vi "Read Value.vi"(8 "error in (no error)":errorcluster, 11 "sfixed32 in":refnum<class "sfixed32.lvclass">) -> (0 "error out":errorcluster, 2 "Value":i32, 3 "sfixed32 out":refnum<class "sfixed32.lvclass">)   [LabVIEW 2020, in "Protobuf RAW.lvlib" / "sfixed32.lvclass"]
uses:
  sfixed32.lvclass
  sfixed32.lvclass/sfixed32.ctl
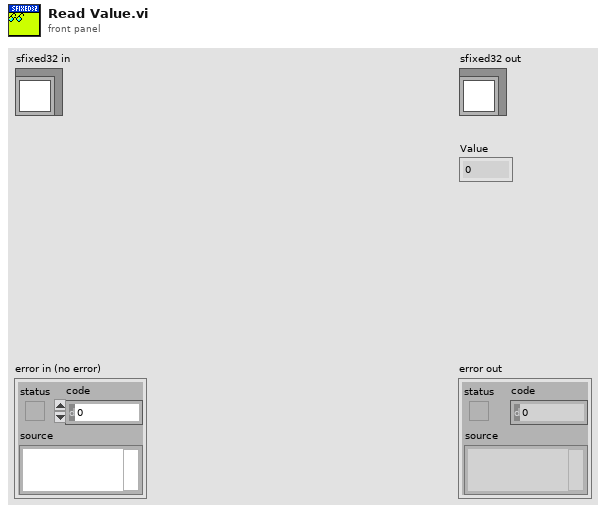
[diagram p1: front panel]
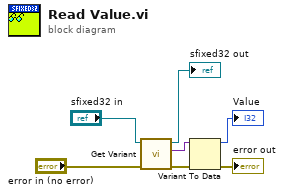
[diagram p0: block diagram]
diagram:
  n1 = call-dynamic "Get Variant.vi"("error in (no error)"="error in (no error)", "Proto Type Common in"="sfixed32 in") -> ("error out"=w6:errorcluster, "Value"=w2:variant, "Proto Type Common out"=→"sfixed32 out":refnum<class "sfixed32.lvclass">)  [unwired: 7 in]
  n2 = Variant To Data(error in=w6, Variant=w2) -> (data=→"Value":i32, error out=→"error out":errorcluster)  [unwired: 1 in]
